vi "Sub_kalman_discrete_model.vi"(11 "KF":T1={"State"=[[1.0], [0.0]], "F state prop matrix"=[[1.0, 0.0], [0.0, 1.0]], "H measure matrix"=[[1.0, 0.0]], "P process cov"=[], "R measure cov"=[], "Q state cov"=[], "T Sample"=0.0, "New Measurement"=0.0, "Measurement Variance"=0.0, "State Variance"=0.0, "Threshold"=0.0, "Initialized"=FALSE}) -> (3 "KF":T1)   [LabVIEW 2021]
uses:
  <vilib>/Analysis/7linalg.llb/Real Matrix Exp.vi
  <vilib>/Analysis/Matrix/Numeric/Absolute Value/Absolute Value - RM.vi
  <vilib>/Analysis/NI_AALBase.lvlib
  <vilib>/Analysis/Matrix/NI_Matrix.lvlib
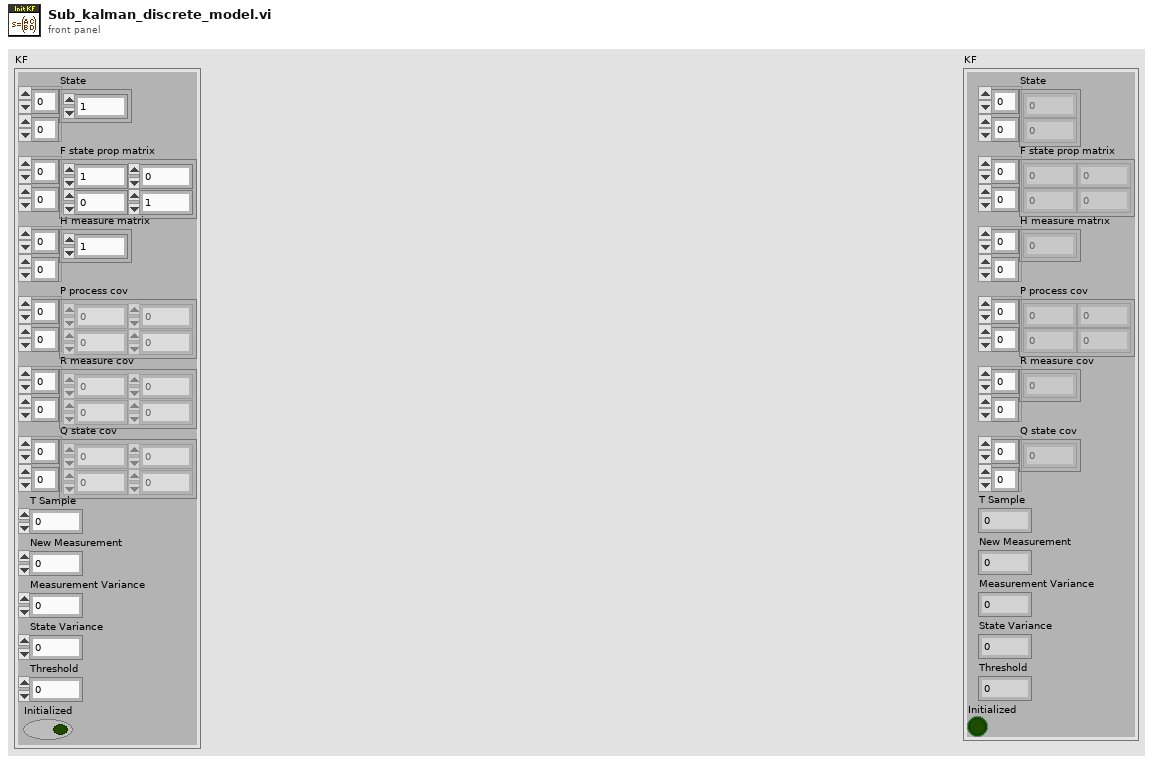
[diagram p1: front panel]
types:
  T1 = cluster{"State":dbl[][], "F state prop matrix":dbl[][], "H measure matrix":dbl[][], "P process cov":dbl[][], "R measure cov":dbl[][], "Q state cov":dbl[][], "T Sample":dbl, "New Measurement":dbl, "Measurement Variance":dbl, "State Variance":dbl, "Threshold":dbl, "Initialized":bool}
  T2 = cluster{"Z hist":dbl[][], "X hist":dbl[][], "A matrix":dbl[][], "C matrix":dbl[][], "P hist":dbl[][], "R matrix":dbl[][], "Q matrix":dbl[][], "T Sample":dbl, "New Measurement":dbl, "Measurement Variance":dbl, "State Variance":dbl}
  T3 = typedef "NI_Matrix.lvlib/RealMatrix.ctl" = dbl[][]
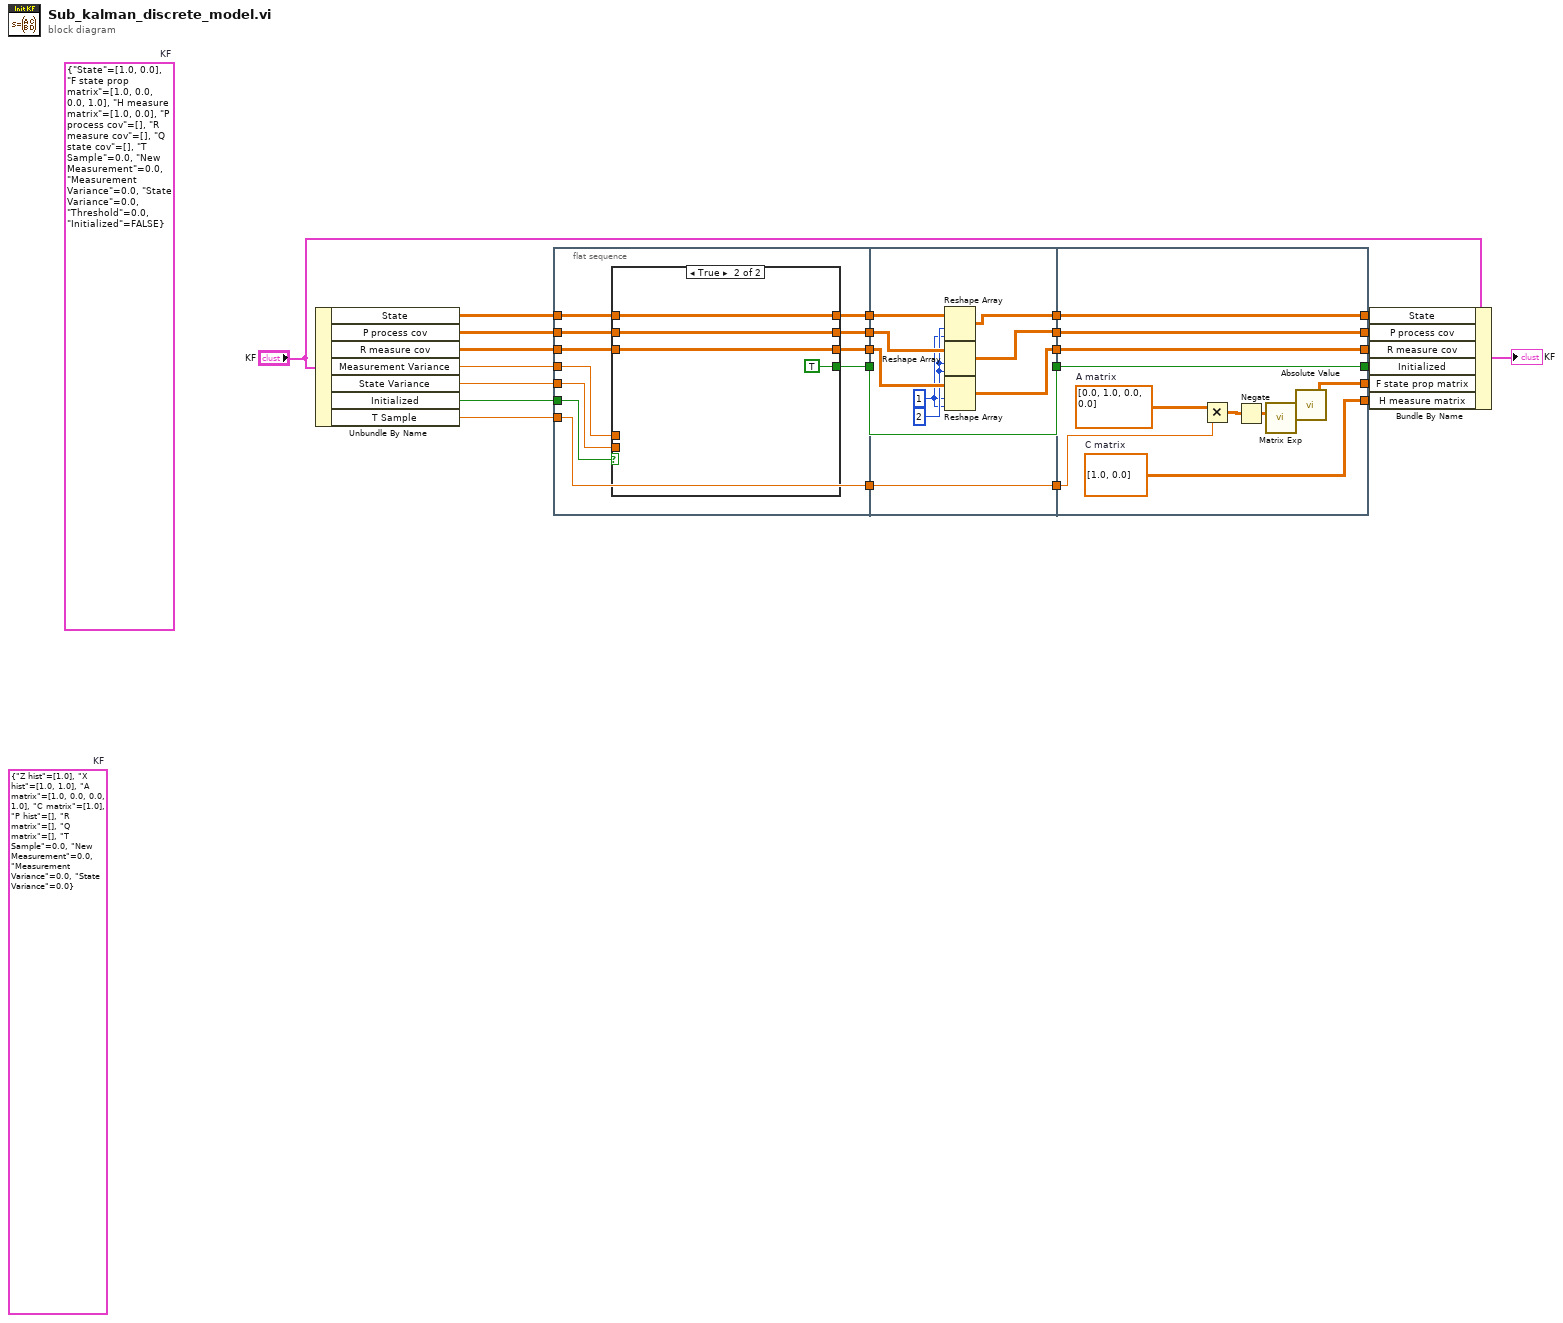
[diagram p0: block diagram]
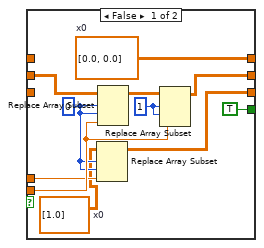
[diagram p2: hidden frame]
diagram:
  (unwired) T1 {"State"=[[1.0], [0.0]], "F state prop matrix"=[[1.0, 0.0], [0.0, 1.0]], "H measure matrix"=[[1.0, 0.0]], "P process cov"=[], "R measure cov"=[], "Q state cov"=[], "T Sample"=0.0, "New Measurement"=0.0, "Measurement Variance"=0.0, "State Variance"=0.0, "Threshold"=0.0, "Initialized"=FALSE}  # KF
  (unwired) T2 {"Z hist"=[[1.0]], "X hist"=[[1.0], [1.0]], "A matrix"=[[1.0, 0.0], [0.0, 1.0]], "C matrix"=[[1.0]], "P hist"=[], "R matrix"=[], "Q matrix"=[], "T Sample"=0.0, "New Measurement"=0.0, "Measurement Variance"=0.0, "State Variance"=0.0}  # KF
  n1 = Unbundle By Name("KF") -> ("State"=w24:dbl[][], "P process cov"=w23:dbl[][], "R measure cov"=w22:dbl[][], "Measurement Variance"=w19:dbl, "State Variance"=w20:dbl, "Initialized"=w21:bool, "T Sample"=w11:dbl)
  n2 = flat-sequence {
    tunnel: w21 -> [w36]
    tunnel: w20 -> [w35]
    tunnel: w19 -> [w34]
    tunnel: w22 -> [w33]
    tunnel: w23 -> [w32]
    tunnel: w24 -> [w31]
    tunnel: [w30] -> w10
    tunnel: [w29] -> w8
    tunnel: [w28] -> w6
    tunnel: [w27] -> w4
    tunnel: w11 -> [w26]
    tunnel: [w26] -> w2
    tunnel: w10 -> [w59]
    tunnel: [w56] -> w9
    tunnel: w8 -> [w58]
    tunnel: [w55] -> w7
    tunnel: w6 -> [w57]
    tunnel: [w54] -> w5
    tunnel: w4 -> [w61]
    tunnel: [w61] -> w3
    tunnel: w2 -> [w60]
    tunnel: [w60] -> w1
    tunnel: [w62] -> w15
    tunnel: [w72] -> w14
    tunnel: w9 -> [w71]
    tunnel: w7 -> [w70]
    tunnel: w5 -> [w69]
    tunnel: [w71] -> w18
    tunnel: [w70] -> w17
    tunnel: [w69] -> w16
    tunnel: w3 -> [w68]
    tunnel: [w68] -> w13
    tunnel: w1 -> [w67]
    frame #0 {
      n3 = case shown="True" w36 {
        tunnel: w35 -> [w47 _]
        tunnel: w34 -> [w42 _]
        tunnel: w33 -> [_ w49]
        tunnel: w32 -> [w45 w50]
        tunnel: w31 -> [_ w51]
        tunnel: [w43 w51] -> w30
        tunnel: [w40 w50] -> w29
        tunnel: [w39 w49] -> w28
        tunnel: [TRUE TRUE] -> w27
        frame False {
          w37 = dbl[][] [[1.0]]  # x0
          w46 = 1 ("disabled index (col)")
          w41 = 0 ("index (row)")
          w43 = dbl[][] [[0.0], [0.0]]  # x0
          n4 = Replace Array Subset(array=w37, new element=w42, index (row)=w41, index (col)=w41) -> (w39:dbl[][])
          n5 = Replace Array Subset(array=w45, new element=w47, index (row)=w41, index (col)=w41) -> (w44:dbl[][])
          n6 = Replace Array Subset(array=w44, new element=w47, index (row)=w46, index (col)=w46) -> (w40:dbl[][])
        }
        frame True {
        }
      }
    }
    frame #1 {
      w53 = 2
      w52 = 1
      n7 = Reshape Array(w59, w53, w52) -> (w56:dbl[][])
      n8 = Reshape Array(w58, w53, w53) -> (w55:dbl[][])
      n9 = Reshape Array(w57, w52, w52) -> (w54:dbl[][])
    }
    frame #2 {
      w64 = dbl[][] [[0.0, 1.0], [0.0, 0.0]]  # A matrix
      w72 = dbl[][] [[1.0, 0.0]]  # C matrix
      n10 = Multiply(x=w64, y=w67) -> (x*y=w65:dbl[][])
      n11 = Negate(x=w65) -> (-x=w66:dbl[][])
      n12 = call-poly <vilib>:"Matrix Exp.vi"("Input Matrix"=w66) -> ("Matrix Exp"=w63:T3)  [unwired: 1 in, 1 out]
      n13 = call-poly <vilib>:"Absolute Value.vi"("Real Matrix A"=w63) -> ("|A|"=w62:T3)
    }
  }
  n14 = Bundle By Name(cluster="KF", "State"=w18, "P process cov"=w17, "R measure cov"=w16, "Initialized"=w13, "F state prop matrix"=w15, "H measure matrix"=w14) -> (→"KF":T1)
